vi "Data Class_1D Str.vi"(5 "삭제?(F)":bool, 9 "대체 문자열":string, 10 "DATA 입력":string[](array[string]), 11 "검색 문자열":string) -> (2 "배열크기":i32, 3 "DATA 출력":string[](array[string]))   [LabVIEW 2020]
panel:
  out "제외 DATA 출력":string[](array[string])
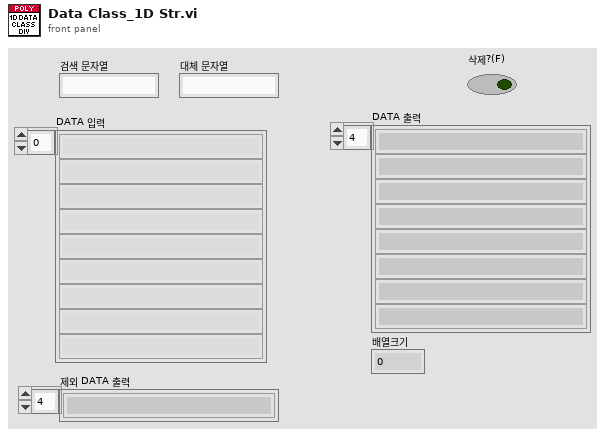
[diagram p1: front panel]
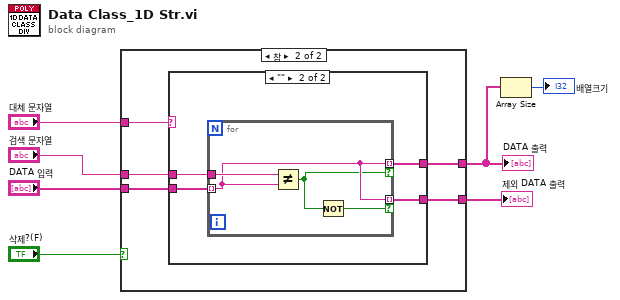
[diagram p0: block diagram]
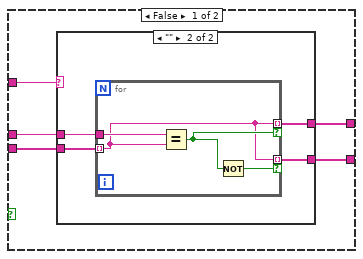
[diagram p2: hidden frame]
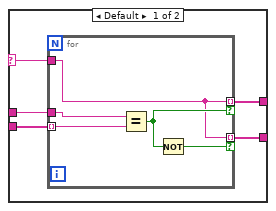
[diagram p3: hidden frame]
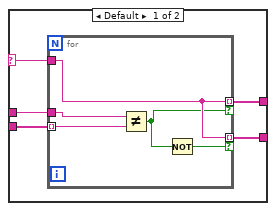
[diagram p4: hidden frame]
diagram:
  n1 = case shown="참" "삭제?(F)" {
    tunnel: [w12 w35] -> w3
    tunnel: "검색 문자열" -> [w11 w34]
    tunnel: "DATA 입력" -> [w10 w33]
    tunnel: "대체 문자열" -> [w9 w32]
    tunnel: [w8 w31] -> w1
    frame False {
      n2 = case shown="\"\"" w9 {
        selector: w9 -> [w14 _]
        tunnel: [w17 w26] -> w12
        tunnel: w11 -> [w16 w25]
        tunnel: w10 -> [w15 w24]
        tunnel: [w13 w23] -> w8
        frame Default {
          n3 = for {
            tunnel: w15 -> [w21] mode=indexing
            tunnel: w16 -> [w22]
            tunnel: [w19] -> w17 mode=indexing if=w20
            tunnel: w14 -> [w19]
            tunnel: [w19] -> w13 mode=indexing if=w18
            n4 = Equal?(x=w22, y=w21) -> (x = y?=w20:bool)
            n5 = Not(x=w20) -> (.not. x?=w18:bool)
          }
        }
        frame "" {
          n6 = for {
            tunnel: w24 -> [w28] mode=indexing
            tunnel: w25 -> [w30]
            tunnel: [w28] -> w26 mode=indexing if=w29
            tunnel: [w28] -> w23 mode=indexing if=w27
            n7 = Equal?(x=w30, y=w28) -> (x = y?=w29:bool)
            n8 = Not(x=w29) -> (.not. x?=w27:bool)
          }
        }
      }
    }
    frame True {
      n9 = case shown="\"\"" w32 {
        selector: w32 -> [w37 _]
        tunnel: [w40 w49] -> w35
        tunnel: w34 -> [w39 w48]
        tunnel: w33 -> [w38 w47]
        tunnel: [w36 w46] -> w31
        frame Default {
          n10 = for {
            tunnel: w38 -> [w44] mode=indexing
            tunnel: w39 -> [w45]
            tunnel: [w43] -> w40 mode=indexing if=w41
            tunnel: w37 -> [w43]
            tunnel: [w43] -> w36 mode=indexing if=w42
            n11 = Not Equal?(x=w45, y=w44) -> (x != y?=w41:bool)
            n12 = Not(x=w41) -> (.not. x?=w42:bool)
          }
        }
        frame "" {
          n13 = for {
            tunnel: w47 -> [w52] mode=indexing
            tunnel: w48 -> [w53]
            tunnel: [w52] -> w49 mode=indexing if=w50
            tunnel: [w52] -> w46 mode=indexing if=w51
            n14 = Not Equal?(x=w53, y=w52) -> (x != y?=w50:bool)
            n15 = Not(x=w50) -> (.not. x?=w51:bool)
          }
        }
      }
    }
  }
  "DATA 출력" <- w3
  "제외 DATA 출력" <- w1
  n16 = Array Size(array=w3) -> (size(s)=→"배열크기":i32)
